vi "Retrieve Measurement Plugin from Server.vi"(8 "error in (no error)":errorcluster, 10 "Measurement Name":string, 11 "Location of Server":string) -> (0 "error out":errorcluster, 3 "Path to Measurement Plugin":path)   [LabVIEW 2016, in "Client Controller.lvlib" / "Client Controller.lvclass"]
uses:
  Client Controller.lvclass
  <vilib>/httpClient/LabVIEWHTTPClient.lvlib
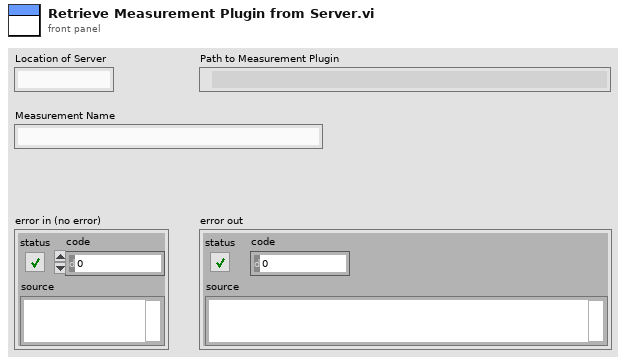
[diagram p1: front panel]
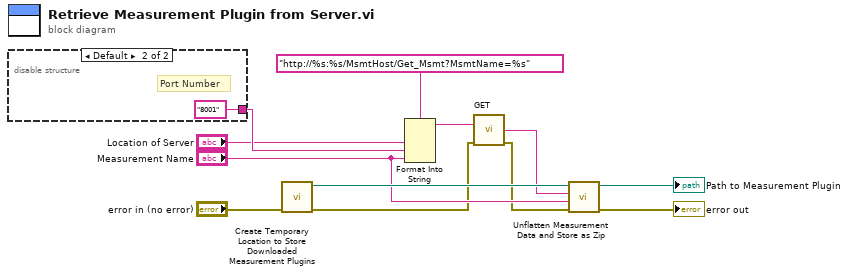
[diagram p0: block diagram]
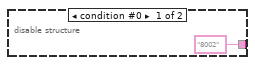
[diagram p2: hidden frame]
diagram:
  n1 = disable-structure shown="Default" {
    disable-tunnel: ["8002" ("input 2") "8001" ("input 2")] -> w11
    frame condition #0 {
    }
    frame condition #1 (active) {
      # "Port Number"
    }
  }
  n2 = call "Create Temporary Location to Store Downloaded Measurement Plugins.vi"("error in (no error)"="error in (no error)") -> ("error out"=w2:errorcluster, "created path"=w12:path)  [unwired: 9 in]
  n3 = Format Into String(format string="http://%s:%s/MsmtHost/Get_Msmt?MsmtName=%s", "Location of Server", w11, "Measurement Name") -> (resulting string=w4:string)  [unwired: 2 in, 1 out]
  n4 = call <vilib>:"GET.vi"("url"=w4, "error in (no error)"=w2) -> ("body"=w3:string, "error out"=w1:errorcluster)  [unwired: 10 in, 2 out]
  n5 = call "Unflatten Measurement Data and Store as Zip.vi"("error in (no error)"=w1, "Measurement Name"="Measurement Name", "Measurement Data"=w3, "Path to Store Measurement"=w12) -> ("error out"=→"error out":errorcluster, "Folder Location"=→"Path to Measurement Plugin":path)  [unwired: 6 in]
